vi "Report_Type.vi"(8 "error in (no error)":errorcluster, 11 "IB_DLL in":refnum<class "IB_DLL.lvclass">) -> (0 "error out":errorcluster, 2 "type":string, 3 "IB_DLL out":refnum<class "IB_DLL.lvclass">)   [LabVIEW 2020, in "IB_DLL.lvclass"]
uses:
  <vilib>/AppBuilder/IB_Classes/Source/Container/Build/DLL/IB_DLL.lvclass
  <vilib>/AppBuilder/IB_Classes/Source/Container/Build/DLL/IB_DLL.lvclass/IB_DLL.ctl
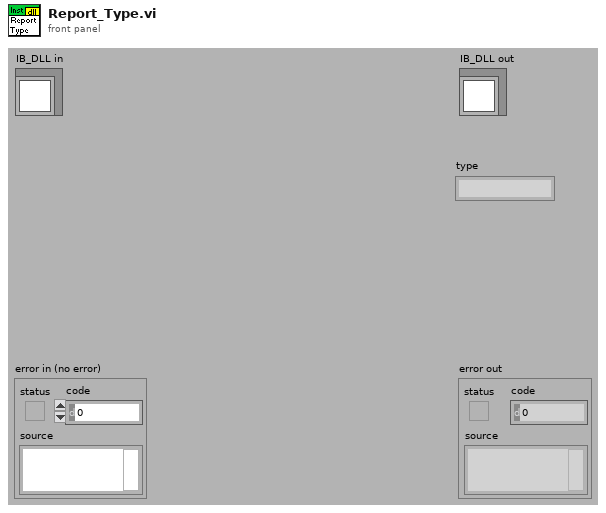
[diagram p1: front panel]
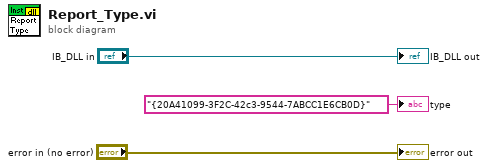
[diagram p0: block diagram]
diagram:
  "error out" <- "error in (no error)"
  "IB_DLL out" <- "IB_DLL in"
  "type" <- "{20A41099-3F2C-42c3-9544-7ABCC1E6CB0D}" ("type")
